vi "Smooth Data.vi"(8 "error in (no error)":errorcluster, 10 "Data Array":dbl[][](array[numeric]), 11 "dt":dbl) -> (0 "error out":errorcluster, 3 "Resampled Array":dbl[][](array[numeric]))   [LabVIEW 2021]
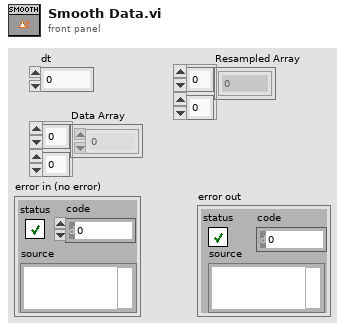
[diagram p1: front panel]
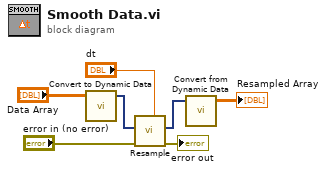
[diagram p0: block diagram]
diagram:
  n1 = call "Convert to Dynamic Data"("2D Array"="Data Array") -> ("Dynamic Data Type"=w3:dynamicdata)  [unwired: 3 in]
  n2 = call "Resample"("dt"="dt", "error in (no error)"="error in (no error)", "Signals"=w3) -> ("error out"=→"error out":errorcluster, "Resampled Signals"=w4:dynamicdata)  [unwired: 6 in, 1 out]
  n3 = call "Convert from Dynamic Data"("Dynamic Data Type"=w4) -> ("Array"=→"Resampled Array":dbl[][])  [unwired: 3 in]
